vi "Load Class Path.vi"(7 "Class Name":string, 8 "error in":errorcluster, 10 "lvlibp path":path, 11 "Configuration in":refnum<class "Configuration.lvclass">) -> (0 "error out":errorcluster, 2 "Class Path":path, 3 "Configuration out":refnum<class "Configuration.lvclass">)   [LabVIEW 2018, in "Configuration.lvlib" / "Configuration.lvclass"]
doc: "This program searches for the class path. It will return a path whether or not a class is bundled into a packed project library. \n\nIf the class is not stored in the folder hierarchy, it will not be able to find the file and will return an error."
uses:
  Configuration.lvclass
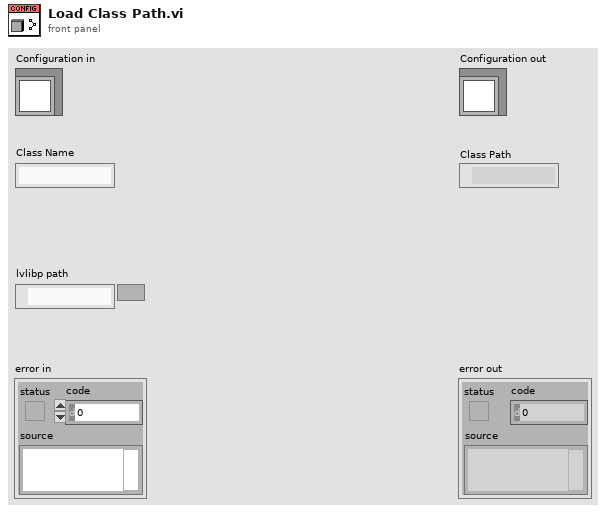
[diagram p1: front panel]
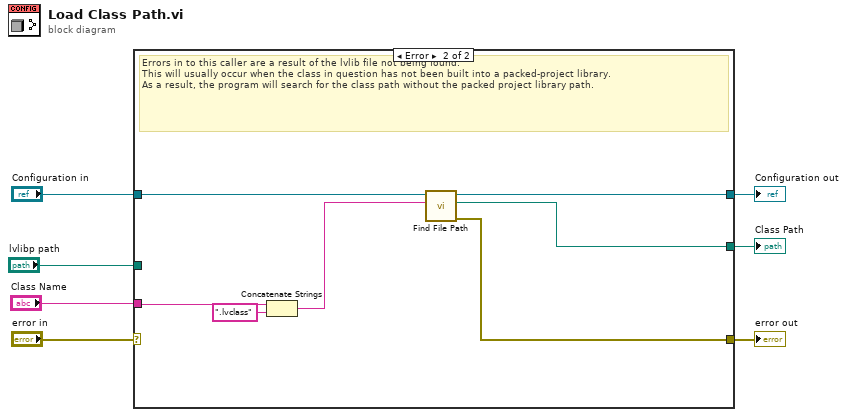
[diagram p0: block diagram]
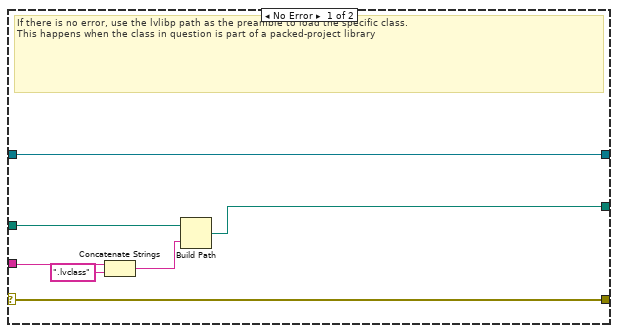
[diagram p2: hidden frame]
diagram:
  n1 = case shown="Error" "error in" {
    selector: "error in" -> [w13 _]
    tunnel: [w13 w17] -> w6
    tunnel: [w14 w18] -> w4
    tunnel: "Configuration in" -> [w14 w19]
    tunnel: "Class Name" -> [w12 w21]
    tunnel: [w8 w16] -> w1
    tunnel: "lvlibp path" -> [w10 _]
    frame No Error {
      # "If there is no error, use the lvlibp path as the preamble to load the specific class.  \nThis happens when the class in question is part of a packed-project library"
      n2 = Concatenate Strings(w12, ".lvclass" ("string")) -> (w9:string)
      n3 = Build Path(base path=w10, name or relative path=w9) -> (appended path=w8:path)
    }
    frame Error {
      # "Errors in to this caller are a result of the lvlib file not being found. \nThis will usually occur when the class in question has not been built into a packed-project library.  \nAs a result, the program will search for the class path without the packed project library path."
      n4 = Concatenate Strings(w21, ".lvclass" ("string")) -> (w15:string)
      n5 = call "Find File Path.vi"("Filename"=w15, "Configuration in"=w19) -> ("error out"=w17:errorcluster, "File Path"=w16:path, "Configuration out"=w18:refnum<class "Configuration.lvclass">)  [unwired: 7 in]
    }
  }
  "error out" <- w6
  "Configuration out" <- w4
  "Class Path" <- w1
